vi "output.vi"(8 "error in":errorcluster, 10 "data table in":T1, 11 "Modbus Slave runtime in":refnum<class "Modbus Slave runtime.lvclass">) -> (0 "error out":errorcluster, 2 "data table out":T1, 3 "Modbus Slave runtime out":refnum<class "Modbus Slave runtime.lvclass">)   [LabVIEW 2013, in "Modbus Slave runtime.lvclass"]
doc: "Provides an interface for writing data to a module at runtime. While this interface performs no operations, a child should provide an override which may write to any open sessions, references, or interfaces.Platypus Framework 1.0.1.65\nNI Systems Engineering - National Instruments"
uses:
  Modbus Slave runtime.lvclass
  <vilib>/NI/Tag Bus/table/data table.ctl
  Modbus Slave runtime.lvclass/Modbus Slave runtime.ctl
  <vilib>/NI/Modbus Library/API/Slave/Modbus Slave.lvclass
  <vilib>/NI/Tag Bus/table/data table.lvlib
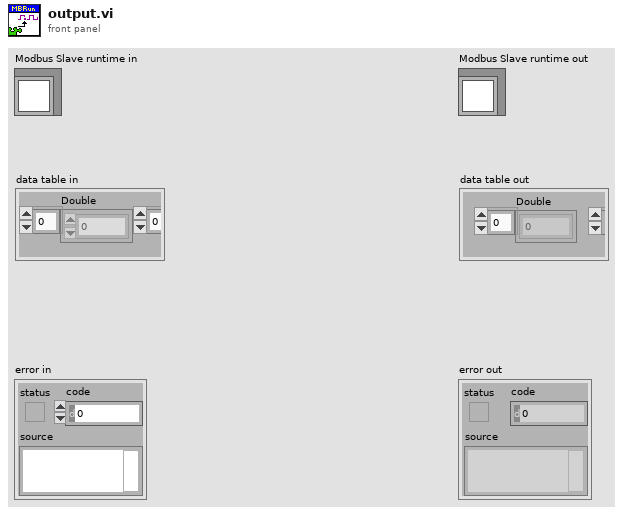
[diagram p1: front panel]
types:
  T1 = typedef "tag bus.lvlib/data table.lvlib/data table.ctl" = cluster{"Double":dbl[], "Single":sgl[], "I64":i64[], "I32":i32[], "I16":i16[], "I8":i8[], "U64":u64[], "U32":u32[], "U16":u16[], "U8":u8[], "Boolean":bool[], "String":string[], "Array of Double":cluster{"DBL Array":dbl[]}[], "Array of Single":cluster{"SGL Array":sgl[]}[], "Array of I64":cluster{"I64 Array":i64[]}[], "Array of I32":cluster{"I32 Array":i32[]}[], "Array of I16":cluster{"I16 Array":i16[]}[], "Array of I8":cluster{"I8 Array":i8[]}[], "Array of U64":cluster{"U64 Array":u64[]}[], "Array of U32":cluster{"U32 Array":u32[]}[], "Array of U16":cluster{"U16 Array":u16[]}[], "Array of U8":cluster{"U8 Array":u8[]}[], "Array of Boolean":cluster{"Boolean Array":bool[]}[], "Array of String":cluster{"String Array":string[]}[]}
  T2 = typedef "Modbus Slave runtime.lvclass/output bulk data access.ctl" = cluster{"modbus type":T3, "start":u16, "length":u16, "maps":T4[], "coils":bool[], "registers":u16[]}
  T3 = typedef "Modbus Module Channel.lvclass/data bank type.ctl" = enum16{"coils", "discrete inputs", "input registers", "holding registers"}
  T4 = typedef "Modbus Slave runtime.lvclass/data mapping elements.ctl" = cluster{"data type":T5, "data index":i32, "element index":i32, "subindex":i32}
  T5 = typedef "tag bus.lvlib/tag descriptor.lvclass/Data Type.ctl" = enum16{"Double", "Single", "I64", "I32", "I16", "I8", "U64", "U32", "U16", "U8", "Boolean", "String", "Array of Double", "Array of Single", "Array of I64", "Array of I32", "Array of I16", "Array of I8", "Array of U64", "Array of U32", "Array of U16", "Array of U8", "Array of Boolean", "Array of String"}
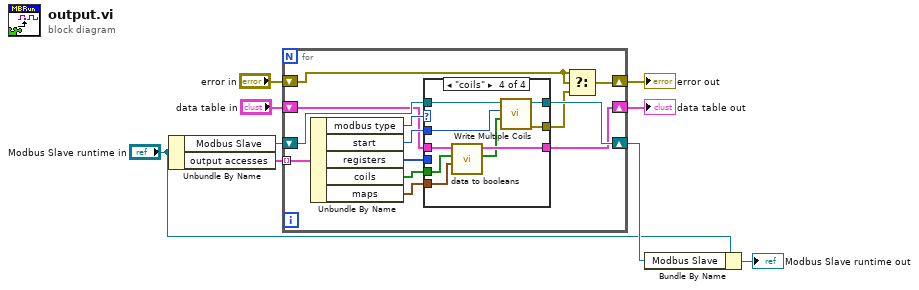
[diagram p0: block diagram]
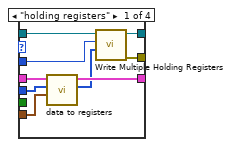
[diagram p2: hidden frame]
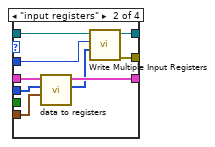
[diagram p3: hidden frame]
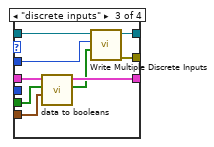
[diagram p4: hidden frame]
diagram:
  n1 = Unbundle By Name("Modbus Slave runtime in") -> ("Modbus Slave"=w9:refnum<class "Modbus Slave.lvclass">, "output accesses"=w7:T2[])
  n2 = for {
    shift-right: [w18] -> w8
    shift-left: w9 -> [w19]
    shift-right: [w21] -> w1
    shift-left: "error in" -> [w22]
    tunnel: w7 -> [w20] mode=indexing
    shift-right: [w11] -> w4
    shift-left: "data table in" -> [w12]
    n3 = Unbundle By Name(w20) -> ("modbus type"=w16:T3, "start"=w15:u16, "registers"=w14:u16[], "coils"=w13:bool[], "maps"=w10:T4[])
    n4 = case shown="\"coils\"" w16 {
      tunnel: w19 -> [w31 w40 w49 w58]
      tunnel: [w30 w39 w48 w57] -> w18
      tunnel: [w28 w37 w46 w55] -> w17
      tunnel: w15 -> [w29 w38 w47 w56]
      tunnel: w14 -> [w27 w36 _ _]
      tunnel: w13 -> [_ _ w44 w52]
      tunnel: w12 -> [w25 w35 w45 w54]
      tunnel: [w24 w34 w43 w51] -> w11
      tunnel: w10 -> [w26 w32 w41 w53]
      frame "holding registers" {
        n5 = call "data to registers.vi"("specifications"=w26, "allocation"=w27, "data table"=w25) -> ("registers"=w23:u16[], "allocation"=w24:T1)  [unwired: 7 in]
        n6 = call-dynamic "Write Multiple Holding Registers.vi"("registers to write"=w23, "starting address"=w29, "Modbus slave in"=w31) -> ("error out"=w28:errorcluster, "Modbus slave out"=w30:refnum<class "Modbus Slave.lvclass">)  [unwired: 7 in]
      }
      frame "input registers" {
        n7 = call "data to registers.vi"("specifications"=w32, "allocation"=w36, "data table"=w35) -> ("registers"=w33:u16[], "allocation"=w34:T1)  [unwired: 7 in]
        n8 = call-dynamic "Write Multiple Input Registers.vi"("input registers to write"=w33, "starting address"=w38, "Modbus slave in"=w40) -> ("error out"=w37:errorcluster, "Modbus slave out"=w39:refnum<class "Modbus Slave.lvclass">)  [unwired: 7 in]
      }
      frame "discrete inputs" {
        n9 = call "data to booleans.vi"("specifications"=w41, "allocation"=w44, "data table"=w45) -> ("registers"=w42:bool[], "allocation"=w43:T1)  [unwired: 7 in]
        n10 = call-dynamic "Write Multiple Discrete Inputs.vi"("discrete inputs to write"=w42, "starting address"=w47, "Modbus slave in"=w49) -> ("error out"=w46:errorcluster, "Modbus slave out"=w48:refnum<class "Modbus Slave.lvclass">)  [unwired: 7 in]
      }
      frame "coils" {
        n11 = call "data to booleans.vi"("specifications"=w53, "allocation"=w52, "data table"=w54) -> ("registers"=w50:bool[], "allocation"=w51:T1)  [unwired: 7 in]
        n12 = call-dynamic "Write Multiple Coils.vi"("coils to write"=w50, "starting address"=w56, "Modbus slave in"=w58) -> ("error out"=w55:errorcluster, "Modbus slave out"=w57:refnum<class "Modbus Slave.lvclass">)  [unwired: 7 in]
      }
    }
    n13 = Select(t=w22, s=w22, f=w17) -> (s? t:f=w21:errorcluster)
  }
  "error out" <- w1
  "data table out" <- w4
  n14 = Bundle By Name(cluster="Modbus Slave runtime in", "Modbus Slave"=w8) -> (→"Modbus Slave runtime out":refnum<class "Modbus Slave runtime.lvclass">)
